vi "LCDIO Get No Of Output Channels.vi"(8 "error in (no error)":errorcluster caption="Fehler (Eingang, kein Fehler)") -> (0 "error out":errorcluster caption="Fehler (Ausgang)", 3 "Output Channel Count":i32)   [LabVIEW 2021, in "labbCAN_DigIO_API.lvlib"]
doc: "LCDIO_Func long LCDIO_CALL LCDIO_GetNoOfOutputChannels();"
uses:
  labbCAN_DigIO_API.lvlib
  labbCAN_DigIO_API.dll
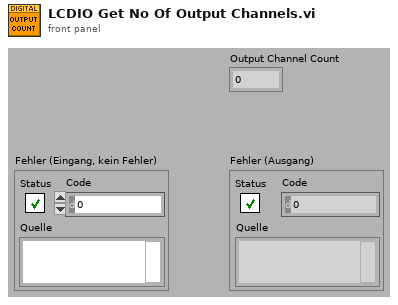
[diagram p1: front panel]
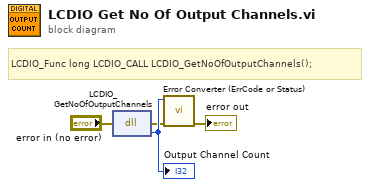
[diagram p0: block diagram]
diagram:
  # "LCDIO_Func long LCDIO_CALL LCDIO_GetNoOfOutputChannels();"
  n1 = dll-call lib="C:/Users/olaja/AppData/Local/CETONI_SDK/labbCAN_DigIO_API.*" fn="LCDIO_GetNoOfOutputChannels"(error in="error in (no error)") -> (error out=w2:errorcluster, w4:i32)  [unwired: 2 in, 1 out]
  "Output Channel Count" <- w4
  n2 = call "Error Converter (ErrCode or Status).vi"("error in (no error)"=w2, "error code"=w4) -> ("error out"=→"error out":errorcluster)  [unwired: 9 in]
